vi "Meas Get Session.vi"(8 "error in":errorcluster, 10 "comment override":string, 11 "record info":T1={"header path"=path "", "group id"=1, "average id"=0, "Time Stamp"=timestamp(0 s since 1904-01-01), "max samples"=0, "first sample"=0, "first smpl [%]"=-1.0, "kill viewer"=FALSE}) -> (0 "error out":errorcluster, 3 "config matrix":string[][](array[string]))   [LabVIEW 2020]
doc: "This will load measurement session and builds formatted matrix of selected parameters for report generation purposes."
uses:
  GUI/GUI Waveform Info.ctl
  octave/infolib/Get 1D String.vi
  octave/infolib/GetI64.vi
  octave/infolib/Get 1D Time Stamp.vi
  octave/infolib/GetString.vi
  octave/infolib/Get 1D I64.vi
  octave/infolib/Get 2D I64.vi
  octave/infolib/infolib.lvlib
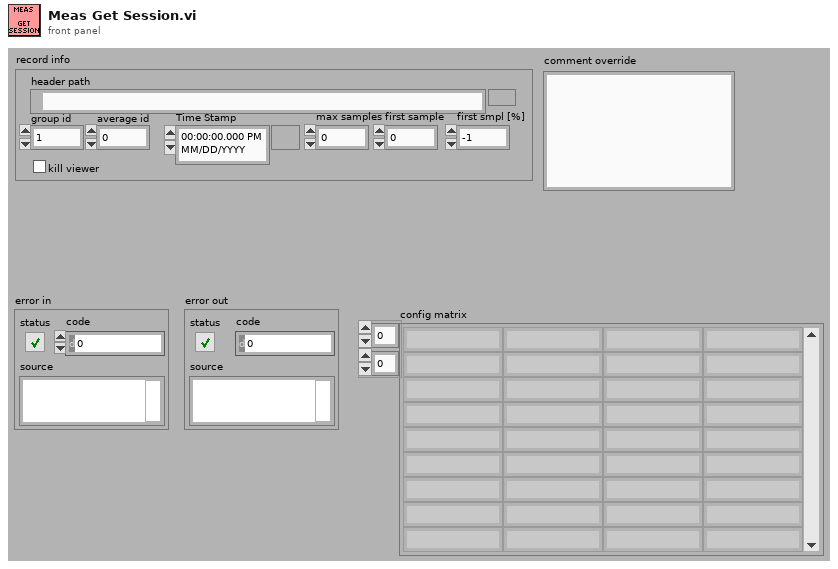
[diagram p1: front panel]
types:
  T1 = typedef "GUI Waveform Info.ctl" = cluster{"header path":path, "group id":i32, "average id":i32, "Time Stamp":timestamp, "max samples":i64, "first sample":i64, "first smpl [%]":dbl, "kill viewer":bool}
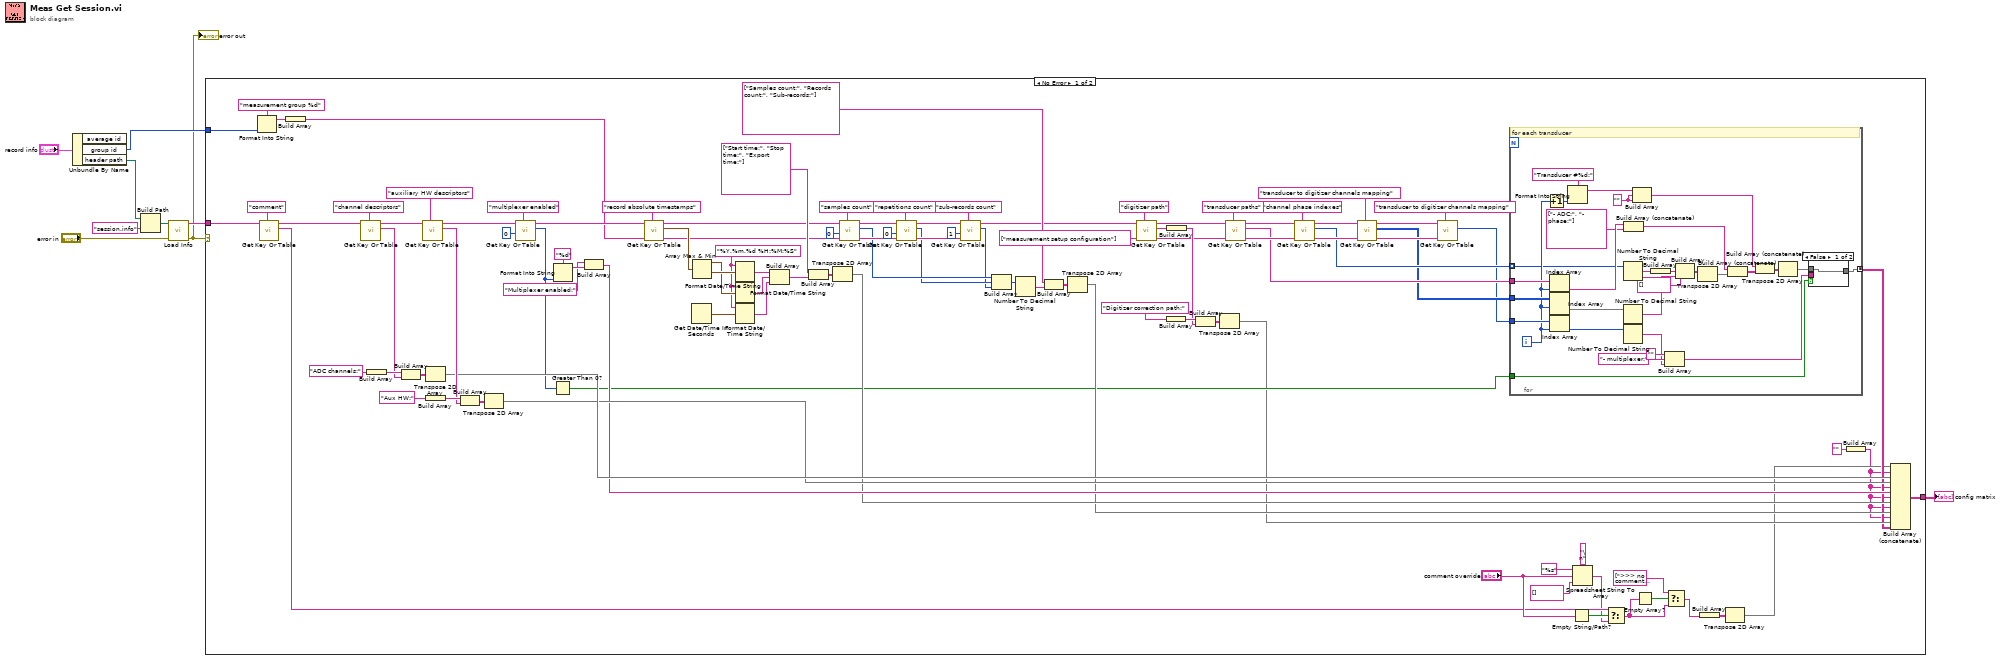
[diagram p0: block diagram]
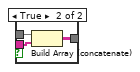
[diagram p2: hidden frame]
diagram:
  n1 = Unbundle By Name("record info") -> ("group id"=w7:i32, "header path"=w3:path)  [unwired: 1 out]
  n2 = Build Path(base path=w3, name or relative path="session.info") -> (appended path=w2:path)
  n3 = call "Load Info.vi"("error in"="error in", "filename"=w2) -> ("error out"=w4:errorcluster, "info data"=w5:string)  [unwired: 8 in]
  "error out" <- w4
  n4 = case shown="No Error" w4 {
    tunnel: w7 -> [w81 _]
    tunnel: [w27 _] -> w6
    tunnel: w5 -> [w22 _]
    frame No Error {
      w89 = "%Y.%m.%d %H:%M:%S" ("format string")
      n5 = Format Into String(format string="measurement group %d", w81) -> (resulting string=w79:string)  [unwired: 2 in, 1 out]
      n6 = call-poly "Get Key Or Table.vi"("key description"="comment", "info data"=w22) -> ("value"=w18:string[], "info data out"=w21:string)  [unwired: 6 in, 2 out]
      n7 = Build Array(w79) -> (w78:string[])
      n8 = call-poly "Get Key Or Table.vi"("key description"="channel descriptors", "info data"=w21) -> ("value"=w106:string[], "info data out"=w112:string)  [unwired: 6 in, 2 out]
      n9 = Build Array("ADC channels:") -> (w107:string[])
      n10 = Build Array(w107, w106) -> (w108:string[][])
      n11 = call-poly "Get Key Or Table.vi"("key description"="auxiliary HW descriptors", "info data"=w112) -> ("value"=w102:string[], "info data out"=w111:string)  [unwired: 6 in, 2 out]
      n12 = Transpose 2D Array(2D array=w108) -> (transposed array=w101:string[][])
      n13 = Build Array("Aux HW:") -> (w105:string[])
      n14 = Build Array(w105, w102) -> (w104:string[][])
      n15 = Transpose 2D Array(2D array=w104) -> (transposed array=w100:string[][])
      n16 = call-poly "Get Key Or Table.vi"("key description"="multiplexer enabled", "numeric"=i64 0, "info data"=w111) -> ("value"=w31:i64, "info data out"=w93:string)  [unwired: 5 in, 2 out]
      n17 = Format Into String(format string="%d", w31) -> (resulting string=w96:string)  [unwired: 2 in, 1 out]
      n18 = Greater Than 0?(x=w31) -> (x > 0?=w30:bool)
      n19 = Build Array("Multiplexer enabled:" ("key description"), w96) -> (w95:string[])
      n20 = call-poly "Get Key Or Table.vi"("key description"="record absolute timestamps", "sections"=w78, "info data"=w93) -> ("sections out"=w75:string[], "value"=w92:timestamp[], "info data out"=w76:string)  [unwired: 5 in, 1 out]
      n21 = Get Date/Time In Seconds() -> (seconds since 1Jan1904=w88:timestamp)
      n22 = Array Max & Min(array=w92) -> (max value=w90:timestamp, min value=w91:timestamp)  [unwired: 2 out]
      n23 = Format Date/Time String(time format string (%c)=w89, seconds (now)=w91) -> (date/time string=w87:string)  [unwired: 1 in]
      n24 = Format Date/Time String(time format string (%c)=w89, seconds (now)=w90) -> (date/time string=w85:string)  [unwired: 1 in]
      n25 = Format Date/Time String(time format string (%c)=w89, seconds (now)=w88) -> (date/time string=w86:string)  [unwired: 1 in]
      n26 = Build Array(w87, w85, w86) -> (w83:string[])
      n27 = Build Array(string[] ["Start time:", "Stop time:", "Export time:"], w83) -> (w84:string[][])
      n28 = Transpose 2D Array(2D array=w84) -> (transposed array=w74:string[][])
      n29 = call-poly "Get Key Or Table.vi"("key description"="samples count", "sections"=w75, "numeric"=i64 0, "info data"=w76) -> ("sections out"=w66:string[], "value"=w61:i64, "info data out"=w67:string)  [unwired: 4 in, 1 out]
      n30 = call-poly "Get Key Or Table.vi"("key description"="repetitions count", "sections"=w66, "numeric"=i64 0, "info data"=w67) -> ("sections out"=w63:string[], "value"=w60:i64, "info data out"=w62:string)  [unwired: 4 in, 1 out]
      n31 = call-poly "Get Key Or Table.vi"("key description"="sub-records count", "sections"=w63, "numeric"=i64 1, "info data"=w62) -> ("value"=w59:i64, "info data out"=w54:string)  [unwired: 4 in, 2 out]
      n32 = Build Array(w61, w60, w59) -> (w58:i64[])
      n33 = Number To Decimal String(number=w58) -> (decimal integer string=w70:string[])  [unwired: 1 in]
      n34 = Build Array(string[] ["Samples count:", "Records count:", "Sub-records:"], w70) -> (w57:string[][])
      n35 = Transpose 2D Array(2D array=w57) -> (transposed array=w56:string[][])
      n36 = call-poly "Get Key Or Table.vi"("key description"="digitizer path", "sections"=string[] ["measurement setup configuration"], "info data"=w54) -> ("sections out"=w45:string[], "value"=w50:string, "info data out"=w46:string)  [unwired: 5 in, 1 out]
      n37 = Build Array("Digitizer correction path:") -> (w53:string[])
      n38 = Build Array(w50) -> (w49:string[])
      n39 = Build Array(w53, w49) -> (w52:string[][])
      n40 = Transpose 2D Array(2D array=w52) -> (transposed array=w29:string[][])
      n41 = call-poly "Get Key Or Table.vi"("key description"="transducer paths", "sections"=w45, "info data"=w46) -> ("sections out"=w42:string[], "value"=w34:string[], "info data out"=w43:string)  [unwired: 5 in, 1 out]
      n42 = call-poly "Get Key Or Table.vi"("key description"="channel phase indexes", "sections"=w42, "info data"=w43) -> ("sections out"=w39:string[], "value"=w35:i64[], "info data out"=w40:string)  [unwired: 5 in, 1 out]
      n43 = call-poly "Get Key Or Table.vi"("key description"="transducer to digitizer channels mapping", "sections"=w39, "info data"=w40) -> ("sections out"=w36:string[], "value"=w33:i64[][], "info data out"=w37:string)  [unwired: 5 in, 1 out]
      n44 = call-poly "Get Key Or Table.vi"("key description"="transducer to digitizer channels mapping", "sections"=w36, "info data"=w37) -> ("value"=w32:i64[])  [unwired: 5 in, 3 out]
      n45 = for {
        tunnel: w35 -> [w135] mode=indexing
        tunnel: w34 -> [w144]
        tunnel: w33 -> [w143]
        tunnel: w32 -> [w142]
        tunnel: [w117] -> w28 mode=concatenating
        tunnel: w30 -> [w115]
        i -> [w141]
        w127 = ""
        # "for each transducer"
        n46 = Increment(x=w141) -> (x+1=w140:i32)
        n47 = Index Array(array=w144, index=w141) -> (element=w138:string)
        n48 = Index Array(array=w143, index (row)=w141) -> (element=w134:i64[])  [unwired: 1 in]
        n49 = Index Array(array=w142, index=w141) -> (element=w133:i64)
        n50 = Format Into String(format string="Transducer #%d:", w140) -> (resulting string=w136:string)  [unwired: 2 in, 1 out]
        n51 = Number To Decimal String(number=w135) -> (decimal integer string=w132:string)  [unwired: 1 in]
        n52 = Number To Decimal String(number=w134) -> (decimal integer string=w131:string[])  [unwired: 1 in]
        n53 = Number To Decimal String(number=w133) -> (decimal integer string=w119:string)  [unwired: 1 in]
        n54 = Build Array (concatenate)(w138, string[] ["- ADC:", "- phase:"]) -> (w128:string[])
        n55 = Build Array(w136, w127, w127) -> (w125:string[])
        n56 = Build Array(w132) -> (w130:string[])
        n57 = Build Array("", "- multiplexer:" ("element"), w119) -> (w116:string[])
        n58 = Build Array(string[] [] ("element"), w130, w131) -> (w129:string[][])
        n59 = Transpose 2D Array(2D array=w129) -> (transposed array=w123:string[][])
        n60 = Build Array (concatenate)(w128, w123) -> (w126:string[][])
        n61 = Build Array (concatenate)(w125, w126) -> (w124:string[][])
        n62 = Transpose 2D Array(2D array=w124) -> (transposed array=w118:string[][])
        n63 = case shown="False" w115 {
          tunnel: w118 -> [w145 w148]
          tunnel: [w145 w147] -> w117
          tunnel: w116 -> [_ w146]
          frame False {
          }
          frame True {
            n64 = Build Array (concatenate)(w148, w146) -> (w147:string[][])
          }
        }
      }
      n65 = Empty String/Path?(string/path="comment override") -> (empty?=w20:bool)
      n66 = Spreadsheet String To Array(delimiter (Tab)="\n", format string="%s", spreadsheet string="comment override", array type (2D Dbl)=string[] []) -> (array=w17:string[])
      n67 = Select(t=w18, s=w20, f=w17) -> (s? t:f=w14:string[])
      n68 = Empty Array?(array=w14) -> (empty?=w15:bool)
      n69 = Select(t=string[] [">>> no comment <<<"], s=w15, f=w14) -> (s? t:f=w13:string[])
      n70 = Build Array(w13) -> (w16:string[][])
      n71 = Transpose 2D Array(2D array=w16) -> (transposed array=w11:string[][])
      n72 = Build Array("") -> (w10:string[])
      n73 = Build Array (concatenate)(w11, w10, w101, w100, w10, w95, w10, w74, w10, w56, w10, w29, w28) -> (w27:string[][])
    }
    frame Error {
    }
  }
  "config matrix" <- w6
